vi "Main - Template.vi"() -> ()   [LabVIEW 2012]
doc: "This is the main user interface for the Theatre Light Control Software."
uses:
  Navistar Library/Controls/TypeDef_Error_Command_enum.ctl
  Navistar Library/Controls/TypeDef - Action - Standard2.ctl
  Navistar Library/Controls/TypeDef - UEvent Selector(Standard).ctl
  Navistar Library/Controls/TypeDef - Queue Selector(Standard).ctl
  Modules/Design Pattern/TypeDef - Template - Queue2 Data Enum.ctl
  Modules/Design Pattern/TypeDef - Template - Queue1 Data Enum.ctl
  Modules/Design Pattern/TypeDef - Template - UEvent Data Enum.ctl
panel:
  in  "Container":enum32{"Page 1"}(tab)
  out "error out":errorcluster
  in  "Stop":bool
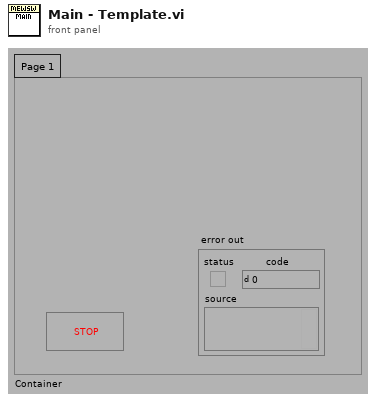
[diagram p1: front panel]
types:
  T1 = typedef "TypeDef - UEvent Selector(Standard).ctl" = enum16{"Create UEvent", "Get UEvent Ref", "Clear UEvent", "Reset UEvent", "Generate U Event"}
  T2 = typedef "TypeDef - Action - Standard2.ctl" = enum16{"Init", "Set", "Get", "Close"}
  T3 = typedef "TypeDef - Queue Selector(Standard).ctl" = enum16{"Create Q", "EnQ", "EnQ at the Opposite", "Flush Q", "Get Q Ref", "Clear Q", "Reset Q"}
  T4 = typedef "TypeDef - Template - Q2 Ref.ctl" = refnum<queue>
  T5 = typedef "TypeDef - Template - Q1 Ref.ctl" = refnum<queue>
  T6 = typedef "TypeDef_Error_Command_enum.ctl" = enum16{"Init", "Check", "Report"}
  T7 = typedef "TypeDef - GPTSV - Queue1 Data Enum.ctl" = enum16{"Queue Enum", "Get Time Data", "Check Time", "Stop"}
  T8 = typedef "TypeDef - Template - UEvent Data Enum.ctl" = enum16{"User Event", "Stop"}
  T9 = typedef "TypeDef - Template - Queue1 Data Enum.ctl" = enum16{"Queue Enum", "Get Time Data", "Check Time", "Stop"}
  T10 = typedef "TypeDef - Template - Queue2 Data Enum.ctl" = enum16{"Queue Enum", "Change RPM", "Stop"}
  T11 = typedef "DSA - UEvent Enum.ctl" = enum16{"User Event", "Stop"}
  T12 = typedef "TypeDef - GPTSV - Queue2 Data Enum.ctl" = enum16{"Queue Enum", "Change RPM", "Stop"}
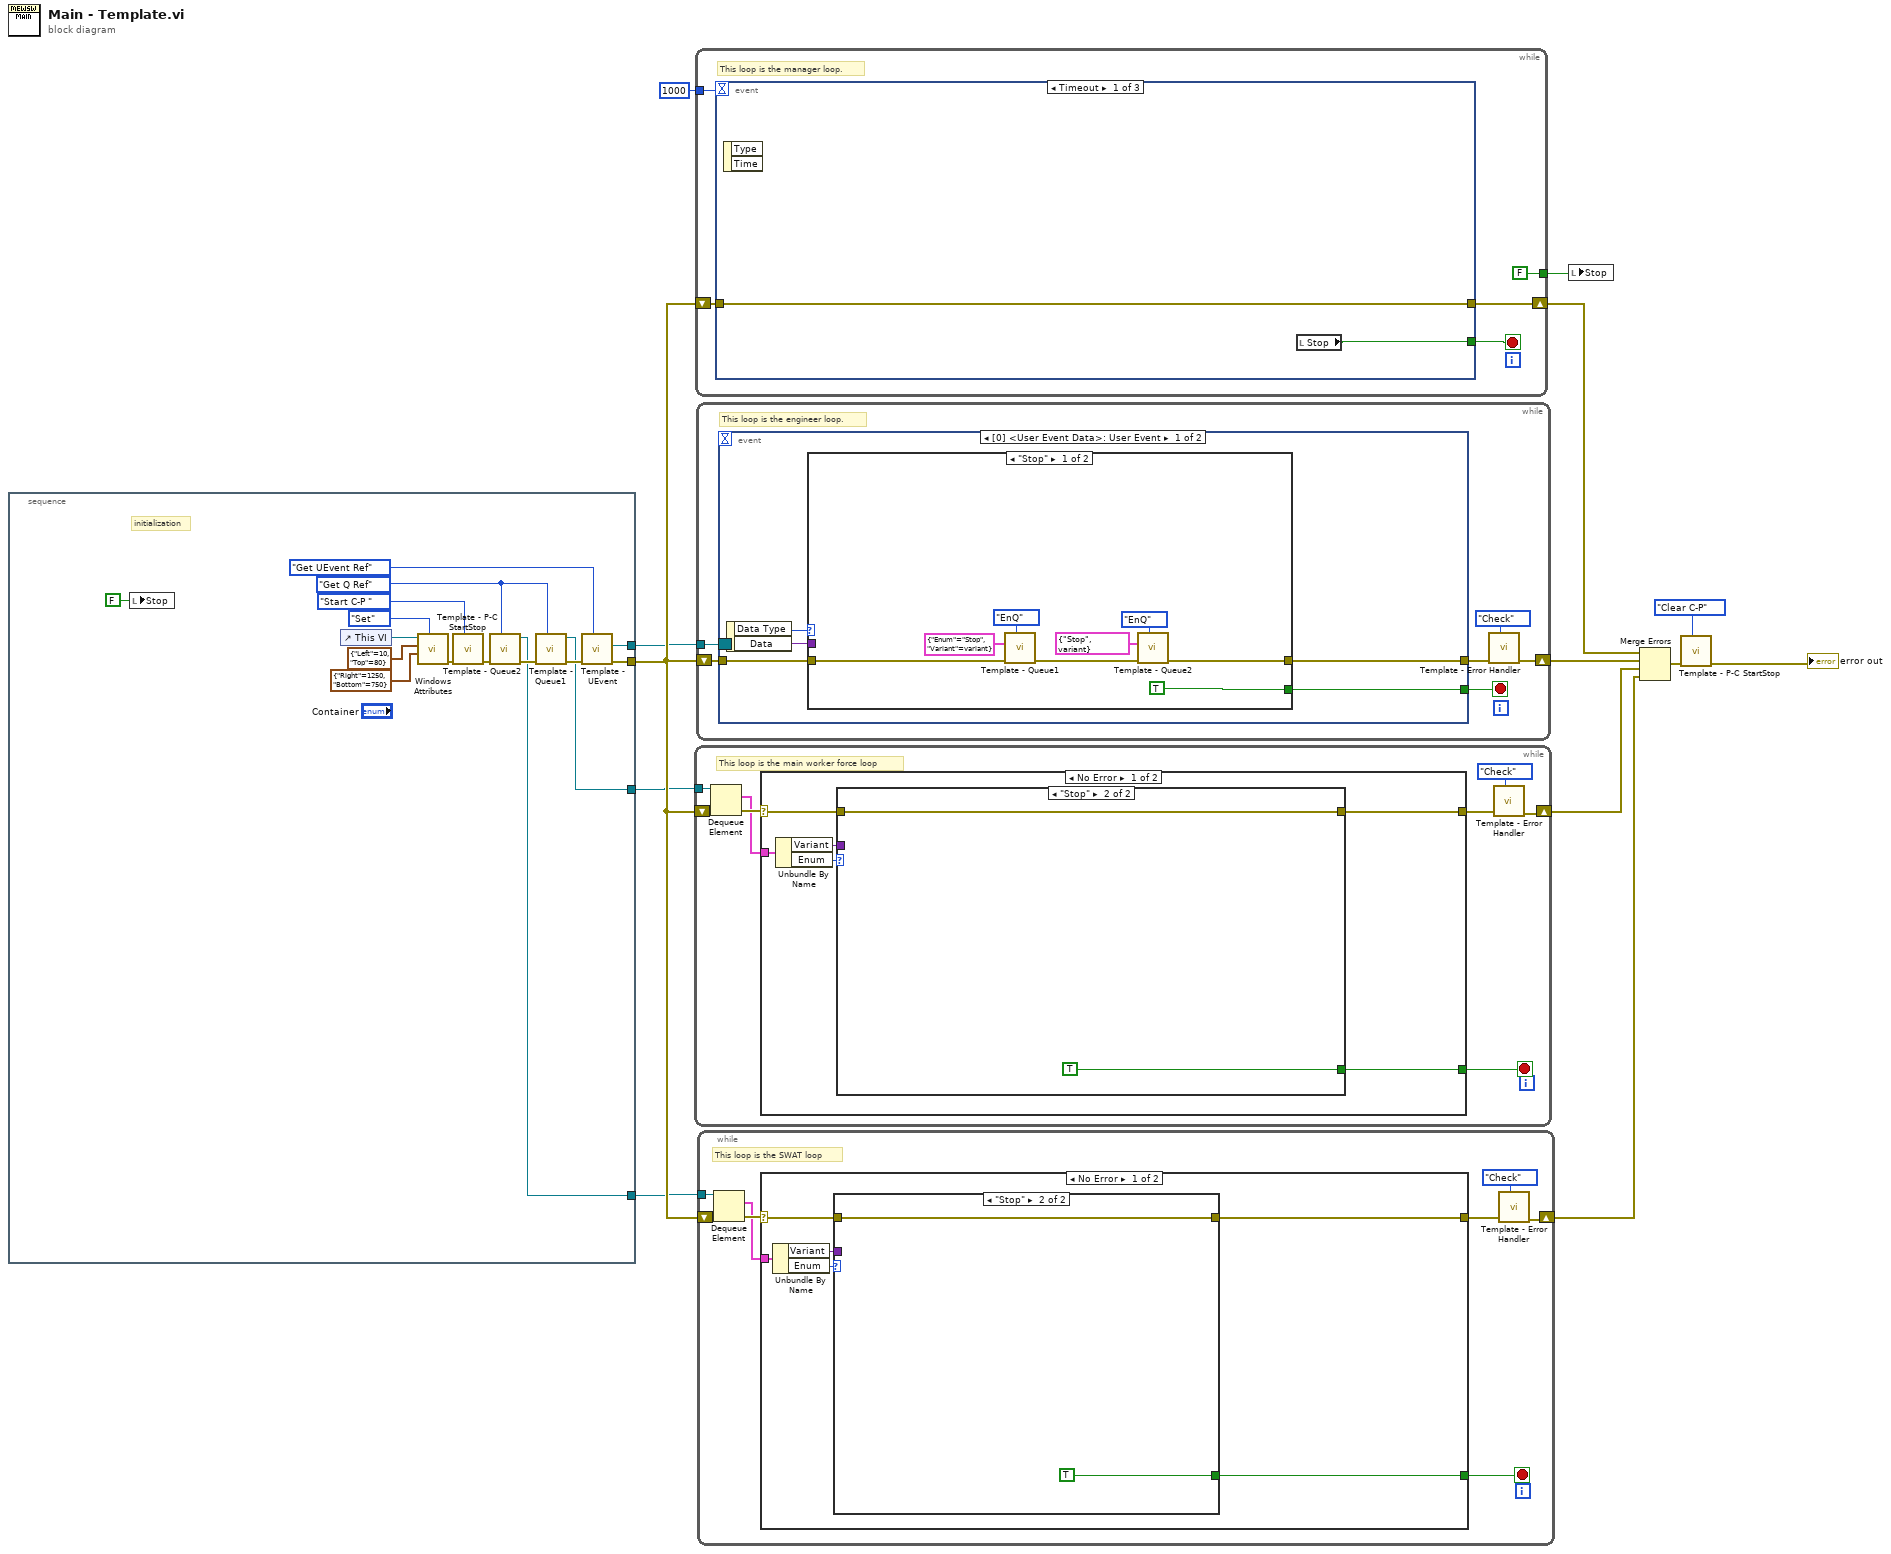
[diagram p0: block diagram]
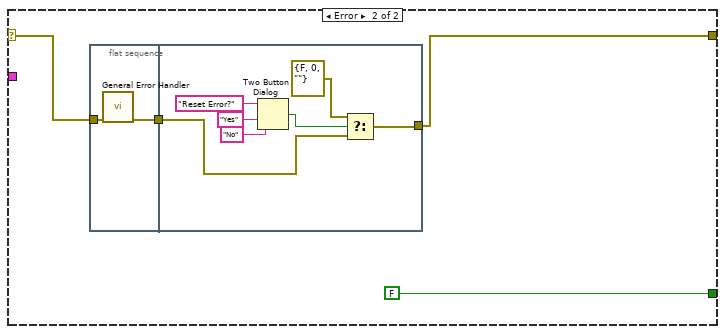
[diagram p3: hidden frame]
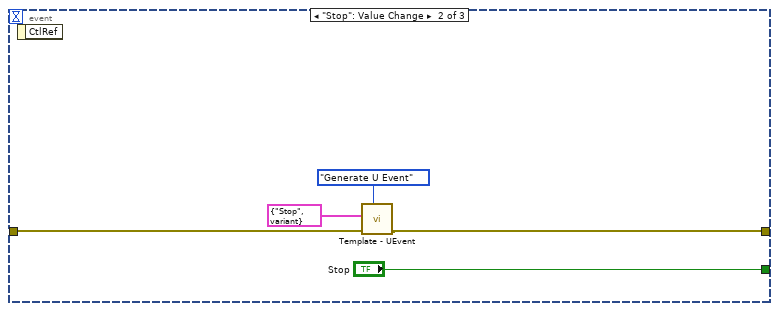
[diagram p4: hidden frame]
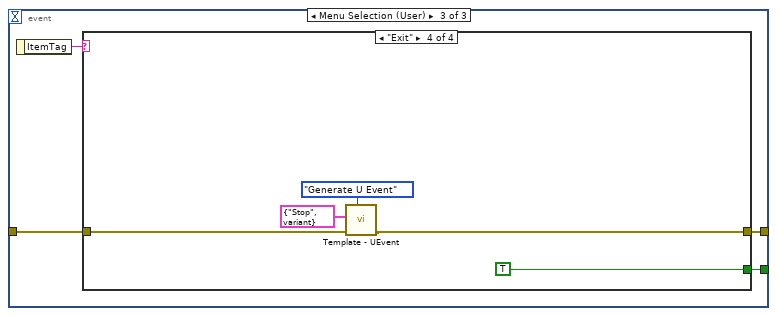
[diagram p5: hidden frame]
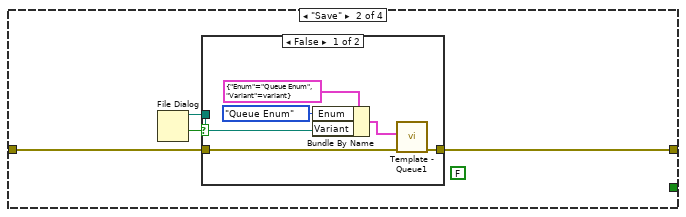
[diagram p7: hidden frame]
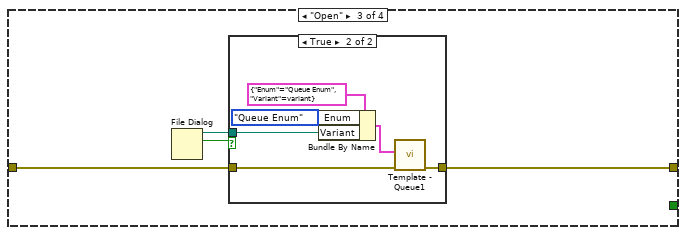
[diagram p9: hidden frame]
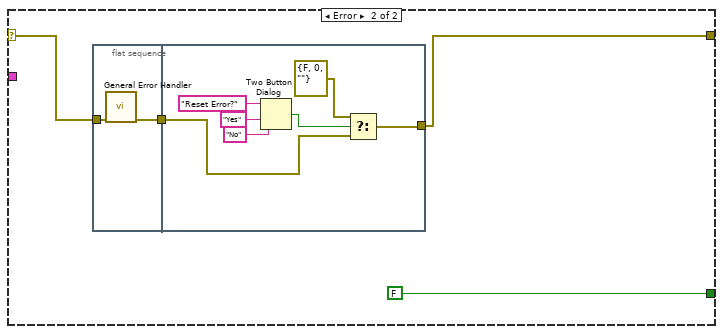
[diagram p12: hidden frame]
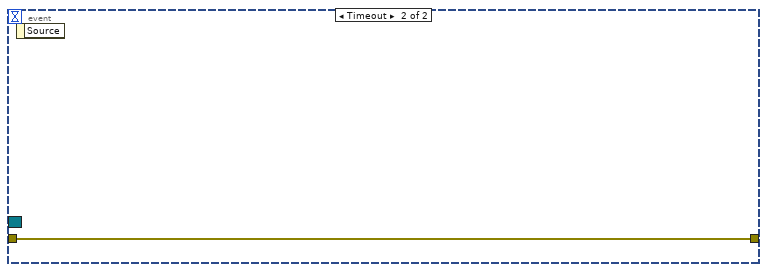
[diagram p14: hidden frame]
diagram:
  n1 = stacked-sequence {
    tunnel: [w23] -> w9
    tunnel: [w22] -> w7
    tunnel: [w20] -> w6
    tunnel: [w17] -> w5
    frame #0 {
      w15 = TypeDef_-_Queue_Selector(Standard)."Get Q Ref" ("Queue Selector")
      # "initialization"
      n2 = local write "Stop"(FALSE ("Stop")) -> ()
      n3 = control-ref of="This VI"() -> (w28:refnum<vi>)
      n4 = call "Windows Attributes.vi"("Action"=TypeDef_-_Action_-_Standard2."Set", "Width/Height"=cluster{"Right":i16, "Bottom":i16} {"Right"=1250, "Bottom"=750} ("Front Panel Window:Panel Bounds"), "Left/Top"=cluster{"Left":i16, "Top":i16} {"Left"=10, "Top"=80} ("Front Panel Window:Panel Bounds"), "This VI"=w28) -> ("error out"=w25:errorcluster)  [unwired: 6 in, 1 out]
      n5 = call "Template - P-C StartStop.vi"("Selector"=enum16{"Start C-P ", "Clear C-P"}."Start C-P ", "error in"=w25) -> ("error out"=w19:errorcluster)  [unwired: 9 in]
      n6 = call "Template - Queue2.vi"("Queue Selector"=w15, "error in (no error)"=w19) -> ("error out"=w18:errorcluster, "Q2 Ref"=w17:T4)  [unwired: 7 in, 1 out]
      n7 = call "Template - Queue1.vi"("Queue Selector"=w15, "error in (no error)"=w18) -> ("error out"=w21:errorcluster, "Q1 Ref"=w20:T5)  [unwired: 7 in, 1 out]
      n8 = call "Template - UEvent.vi"("Event Selector"=TypeDef_-_UEvent_Selector(Standard)."Get UEvent Ref", "error in (no error)"=w21) -> ("error out"=w23:errorcluster, "Event Reg Refnum"=w22:refnum<event-registration>)  [unwired: 7 in, 1 out]
    }
  }
  n9 = while {
    shift-right: [w33] -> w12
    shift-left: w9 -> [w30]
    tunnel: w6 -> [w31]
    stop <- w37 stop-if-true
    # "This loop is the main worker force loop"
    n10 = Dequeue Element(queue=w31, error in (no error)=w30) -> (element=w35:cluster{"Enum":T7, "Variant":variant}, error out=w36:errorcluster)  [unwired: 1 in, 2 out]
    n11 = case shown="No Error" w36 {
      selector: w36 -> [w39 w49]
      tunnel: w35 -> [w43 _]
      tunnel: [w41 FALSE] -> w37
      tunnel: [w38 w47] -> w34
      frame No Error {
        n12 = Unbundle By Name(w43) -> ("Variant"=w40:variant, "Enum"=w42:T7)
        n13 = case shown="\"Stop\"" w42 {
          tunnel: [_ TRUE] -> w41
          tunnel: w40 -> [_ _]
          tunnel: w39 -> [w44 w45]
          tunnel: [w44 w45] -> w38
          frame "Queue Enum", Default {
          }
          frame "Stop" {
          }
        }
      }
      frame Error {
        n14 = flat-sequence {
          tunnel: w49 -> [w52]
          tunnel: [w51] -> w48
          tunnel: w48 -> [w55]
          tunnel: [w53] -> w47
          frame #0 {
            n15 = call <vilib>:"General Error Handler.vi"("error in (no error)"=w52) -> ("error out"=w51:errorcluster)  [unwired: 10 in, 4 out]
          }
          frame #1 {
            n16 = Two Button Dialog(message="Reset Error?", 1:"No" ("F button name (\"Cancel\")"), 2:"Yes" ("T button name (\"OK\")")) -> (T button?=w56:bool)
            n17 = Select(t=errorcluster {"status"=FALSE, "code"=0, "source"=""}, s=w56, f=w55) -> (s? t:f=w53:errorcluster)
          }
        }
      }
    }
    n18 = call "Template - Error Handler.vi"("Command (Check for Error)"=TypeDef_Error_Command_enum."Check", "error in (no error)"=w34) -> ("error out"=w33:errorcluster)  [unwired: 9 in]
  }
  n19 = while {
    shift-right: [w62] -> w3
    shift-left: w9 -> [w63]
    tunnel: 1000 -> [w61]
    tunnel: [FALSE ("Stop")] -> w1
    stop <- w64 stop-if-true
    # "This loop is the manager loop."
    n20 = event shown="[0] Timeout" {
      selector: _ -> [_ _ _]
      dyn-events: _ -> [_ _ _]
      timeout: w61 -> [_ _ _]
      tunnel: [w65 "Stop" w72] -> w64
      tunnel: w63 -> [w66 w68 w74]
      tunnel: [w66 w67 w73] -> w62
      event Timeout {
        n21 = event-data() -> ()  [unwired: 1 in, 2 out]
        n22 = local read "Stop"() -> (w65:bool)
      }
      event "Stop": Value Change {
        n23 = event-data() -> ()  [unwired: 1 in, 1 out]
        n24 = call "Template - UEvent.vi"("Event Selector"=TypeDef_-_UEvent_Selector(Standard)."Generate U Event", "error in (no error)"=w68, "User Event Data"=cluster{"Data Type":T8, "Data":variant} {"Data Type"=enum."Stop", "Data"=variant}) -> ("error out"=w67:errorcluster)  [unwired: 6 in, 2 out]
      }
      event Menu Selection (User) {
        n25 = event-data() -> ("ItemTag"=w75:string)  [unwired: 1 in]
        n26 = case shown="\"Exit\"" w75 {
          tunnel: w74 -> [w76 w80 w91 w102]
          tunnel: [w76 w79 w90 w101] -> w73
          tunnel: [_ _ _ TRUE] -> w72
          frame "False", Default {
          }
          frame "Save" {
            (unwired) FALSE
            n27 = File Dialog() -> (1:w78:bool, 3:w77:path)  [unwired: 7 in, 2 out]
            n28 = case shown="False" w78 {
              tunnel: w80 -> [w83 w87]
              tunnel: [w82 w87] -> w79
              tunnel: w77 -> [w84 _]
              frame False {
                n29 = Bundle By Name(cluster=cluster{"Enum":T9, "Variant":variant} {"Enum"=enum."Queue Enum", "Variant"=variant} ("Cluster"), "Enum"=TypeDef_-_Template_-_Queue1_Data_Enum."Queue Enum", "Variant"=w84) -> (w81:cluster{"Enum":T9, "Variant":variant})
                n30 = call "Template - Queue1.vi"("error in (no error)"=w83, "Queue1 Data"=w81) -> ("error out"=w82:errorcluster)  [unwired: 7 in, 2 out]
              }
              frame True {
              }
            }
          }
          frame "Open" {
            n31 = File Dialog() -> (2:w88:bool, 3:w89:path)  [unwired: 7 in, 2 out]
            n32 = case shown="True" w88 {
              tunnel: w91 -> [w92 w95]
              tunnel: [w92 w94] -> w90
              tunnel: w89 -> [_ w96]
              frame False {
              }
              frame True {
                n33 = Bundle By Name(cluster=cluster{"Enum":T9, "Variant":variant} {"Enum"=enum."Queue Enum", "Variant"=variant} ("Cluster"), "Enum"=TypeDef_-_Template_-_Queue1_Data_Enum."Queue Enum", "Variant"=w96) -> (w93:cluster{"Enum":T9, "Variant":variant})
                n34 = call "Template - Queue1.vi"("error in (no error)"=w95, "Queue1 Data"=w93) -> ("error out"=w94:errorcluster)  [unwired: 7 in, 2 out]
              }
            }
          }
          frame "Exit" {
            n35 = call "Template - UEvent.vi"("Event Selector"=TypeDef_-_UEvent_Selector(Standard)."Generate U Event", "error in (no error)"=w102, "User Event Data"=cluster{"Data Type":T8, "Data":variant} {"Data Type"=enum."Stop", "Data"=variant}) -> ("error out"=w101:errorcluster)  [unwired: 6 in, 2 out]
          }
        }
      }
    }
  }
  n36 = while {
    shift-right: [w107] -> w13
    shift-left: w9 -> [w104]
    tunnel: w7 -> [w105]
    stop <- w109 stop-if-true
    # "This loop is the engineer loop."
    n37 = event shown="[0] <User Event Data>: User Event" {
      selector: w105 -> [_ _]
      dyn-events: _ -> [_ _]
      timeout: _ -> [_ _]
      tunnel: w104 -> [w112 w124]
      tunnel: [w111 w124] -> w108
      tunnel: [w110 _] -> w109
      event User Event {
        n38 = event-data() -> ("Data Type"=w114:T11, "Data"=w113:variant)  [unwired: 1 in]
        n39 = case shown="\"Stop\"" w114 {
          tunnel: w113 -> [_ _]
          tunnel: w112 -> [w121 w123]
          tunnel: [w119 w123] -> w111
          tunnel: [TRUE ("Stop") _] -> w110
          frame "Stop" {
            n40 = call "Template - Queue1.vi"("Queue Selector"=TypeDef_-_Queue_Selector(Standard)."EnQ", "error in (no error)"=w121, "Queue1 Data"=cluster{"Enum":T9, "Variant":variant} {"Enum"=enum."Stop", "Variant"=variant}) -> ("error out"=w120:errorcluster)  [unwired: 6 in, 2 out]
            n41 = call "Template - Queue2.vi"("Queue Selector"=TypeDef_-_Queue_Selector(Standard)."EnQ", "error in (no error)"=w120, "Queue Data"=cluster{"Enum":T10, "Variant":variant} {"Enum"=enum."Stop", "Variant"=variant}) -> ("error out"=w119:errorcluster)  [unwired: 6 in, 2 out]
          }
          frame "User Event" {
          }
        }
      }
      event Timeout {
        n42 = event-data() -> ()  [unwired: 1 in, 1 out]
      }
    }
    n43 = call "Template - Error Handler.vi"("Command (Check for Error)"=TypeDef_Error_Command_enum."Check", "error in (no error)"=w108) -> ("error out"=w107:errorcluster)  [unwired: 9 in]
  }
  n44 = while {
    shift-right: [w128] -> w8
    shift-left: w9 -> [w125]
    tunnel: w5 -> [w126]
    stop <- w132 stop-if-true
    # "This loop is the SWAT loop"
    n45 = Dequeue Element(queue=w126, error in (no error)=w125) -> (element=w130:cluster{"Enum":T12, "Variant":variant}, error out=w131:errorcluster)  [unwired: 1 in, 2 out]
    n46 = case shown="No Error" w131 {
      selector: w131 -> [w134 w144]
      tunnel: w130 -> [w138 _]
      tunnel: [w136 FALSE] -> w132
      tunnel: [w133 w142] -> w129
      frame No Error {
        n47 = Unbundle By Name(w138) -> ("Variant"=w135:variant, "Enum"=w137:T12)
        n48 = case shown="\"Stop\"" w137 {
          tunnel: [_ TRUE] -> w136
          tunnel: w135 -> [_ _]
          tunnel: w134 -> [w139 w140]
          tunnel: [w139 w140] -> w133
          frame "Queue Enum", Default {
          }
          frame "Stop" {
          }
        }
      }
      frame Error {
        n49 = flat-sequence {
          tunnel: w144 -> [w147]
          tunnel: [w146] -> w143
          tunnel: w143 -> [w150]
          tunnel: [w148] -> w142
          frame #0 {
            n50 = call <vilib>:"General Error Handler.vi"("error in (no error)"=w147) -> ("error out"=w146:errorcluster)  [unwired: 10 in, 4 out]
          }
          frame #1 {
            n51 = Two Button Dialog(message="Reset Error?", 1:"No" ("F button name (\"Cancel\")"), 2:"Yes" ("T button name (\"OK\")")) -> (T button?=w151:bool)
            n52 = Select(t=errorcluster {"status"=FALSE, "code"=0, "source"=""}, s=w151, f=w150) -> (s? t:f=w148:errorcluster)
          }
        }
      }
    }
    n53 = call "Template - Error Handler.vi"("Command (Check for Error)"=TypeDef_Error_Command_enum."Check", "error in (no error)"=w129) -> ("error out"=w128:errorcluster)  [unwired: 9 in]
  }
  n54 = local write "Stop"(w1) -> ()
  n55 = Merge Errors(w3, w13, w12, w8) -> (w11:errorcluster)
  n56 = call "Template - P-C StartStop.vi"("Selector"=enum16{"Start C-P ", "Clear C-P"}."Clear C-P", "error in"=w11) -> ("error out"=→"error out":errorcluster)  [unwired: 9 in]
